vi "REP.vi"() -> ()   [LabVIEW 2018]
uses:
  RxTx/RxTx.lvclass
  Channel Rep/Channel Rep.lvclass
  C:/Users/Denis/Desktop/communication-manager/communication-manager/Communication Channel/Communication Channel.lvclass
  <vilib>/addons/zeromq/zmq_context.lvclass
  Communication Channel/Communication Channel.lvclass
panel:
  in  "Channel Rep.lvclass":refnum<class "Channel Rep.lvclass">
  out "error out":errorcluster
  in  "RxTx in":refnum<class "RxTx.lvclass">
  in  "Stop App":bool
  # "REPLY example"
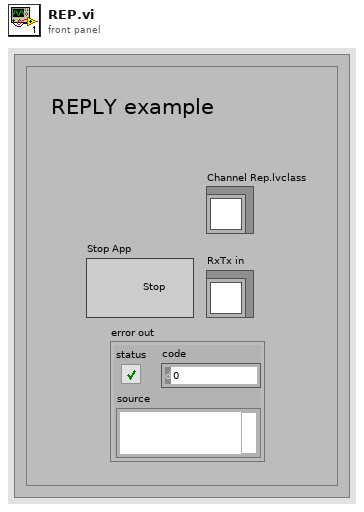
[diagram p1: front panel]
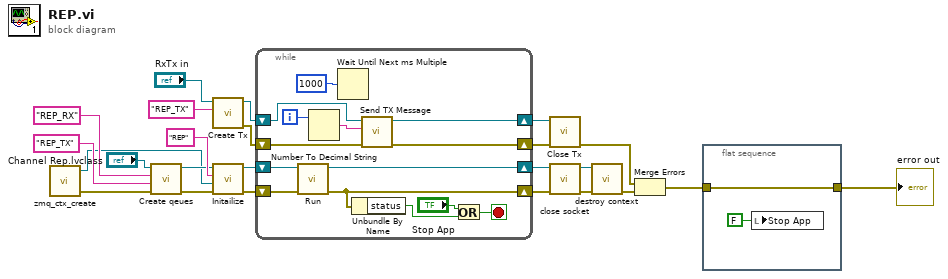
[diagram p0: block diagram]
diagram:
  n1 = call <vilib>:"zmq_ctx_create.vi"() -> ("error out"=w24:errorcluster, "context out"=w6:refnum<class "zmq_context.lvclass">)  [unwired: 4 in]
  n2 = call "Create qeues.vi"("error in (no error)"=w24, "name qeue Tx"="REP_TX" ("name qeue Rx"), "name qeue Rx"="REP_RX", "Communication Channel in"="Channel Rep.lvclass") -> ("error out"=w17:errorcluster, "Communication Channel out"=w18:refnum<class "Channel Rep.lvclass">)  [unwired: 6 in]
  n3 = call "Create Tx.vi"("Writer Name"="REP_TX", "RxTx in"="RxTx in") -> ("error out"=w13:errorcluster, "RxTx out"=w14:refnum<class "RxTx.lvclass">)  [unwired: 8 in]
  n4 = call-dynamic "Initailize.vi"("error in (no error)"=w17, "zeromq.lvlib:ZeroMQ Context"=w6, "Name"="REP", "Channel Pub in"=w18) -> ("error out"=w22:errorcluster, "Channel Pub out"=w23:refnum<class "Channel Rep.lvclass">)  [unwired: 6 in]
  n5 = while {
    shift-right: [w36] -> w20
    shift-left: w23 -> [w38]
    shift-right: [w28] -> w19
    shift-left: w22 -> [w37]
    shift-right: [w33] -> w11
    shift-left: w14 -> [w35]
    shift-right: [w32] -> w10
    shift-left: w13 -> [w34]
    i -> [w31]
    stop <- w25 stop-if-true
    n6 = call-dynamic "Run.vi"("error in (no error)"=w37, "Channel Rep in"=w38) -> ("error out"=w28:errorcluster, "Channel Rep out"=w36:refnum<class "Channel Rep.lvclass">)  [unwired: 8 in]
    n7 = Number To Decimal String(number=w31) -> (decimal integer string=w30:string)  [unwired: 1 in]
    n8 = Wait Until Next ms Multiple(millisecond multiple=u32 1000) -> ()  [unwired: 1 out]
    n9 = Unbundle By Name(w28) -> ("status"=w27:bool)
    n10 = call "Send TX Message.vi"("error in (no error)"=w34, "message"=w30, "RxTx in"=w35) -> ("error out"=w32:errorcluster, "RxTx out"=w33:refnum<class "RxTx.lvclass">)  [unwired: 7 in]
    n11 = Or(x="Stop App", y=w27) -> (x .or. y?=w25:bool)
  }
  n12 = call "Close Tx.vi"("error in (no error)"=w10, "RxTx in"=w11) -> ("error out"=w5:errorcluster)  [unwired: 8 in, 1 out]
  n13 = call "close socket.vi"("error in (no error)"=w19, "Communication Channel in"=w20) -> ("error out"=w8:errorcluster, "Communication Channel out"=w7:refnum<class "Channel Rep.lvclass">)  [unwired: 8 in]
  n14 = call "destroy context.vi"("error in (no error)"=w8, "Communication Channel in"=w7) -> ("error out"=w4:errorcluster)  [unwired: 8 in, 1 out]
  n15 = Merge Errors(w5, w4) -> (w3:errorcluster)
  n16 = flat-sequence {
    tunnel: w3 -> [w40]
    tunnel: [w40] -> w2
    frame #0 {
      n17 = local write "Stop App"(FALSE ("Stop App")) -> ()
    }
  }
  "error out" <- w2
